vi "PathPlanner_Waypoint_AutoCtrlDistFactor.vi"() -> (3 "AUTO_CONTROL_DISTANCE_FACTOR":dbl)   [LabVIEW 2019, in "PathPlanner24.lvlib"]
doc: "The X size or length of the current field in meters\n\nInput:\n -- <none>\n\nOutputs:\n -- FieldSizeX -- X length of field (meters)"
uses:
  PathPlanner24.lvlib
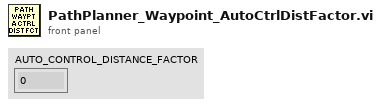
[diagram p1: front panel]
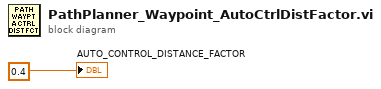
[diagram p0: block diagram]
diagram:
  "AUTO_CONTROL_DISTANCE_FACTOR" <- 0.4 ("Feet")
